vi "SetGetTestClass.vi"(7 "Set? (F)":bool, 11 "TestBase.lvclass":refnum<class "TestBase.lvclass">) -> (3 "TestBase.lvclass":refnum<class "TestBase.lvclass">)   [LabVIEW 2014, in "TestBase.lvclass"]
uses:
  TestBase.lvclass
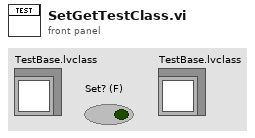
[diagram p1: front panel]
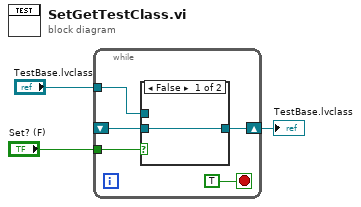
[diagram p0: block diagram]
diagram:
  n1 = while {
    tunnel: "Set? (F)" -> [w8]
    tunnel: "TestBase.lvclass" -> [w7]
    shift-right: [w6] -> w1
    shift-left: _ -> [w5]
    stop <- TRUE stop-if-true
    n2 = case shown="False" w8 {
      tunnel: w7 -> [_ w10]
      tunnel: [w9 w10] -> w6
      tunnel: w5 -> [w9 _]
      frame False {
      }
      frame True {
      }
    }
  }
  "TestBase.lvclass" <- w1
